vi "Type Panel Events.vi"(11 "ColumnPanel":refnum<class "ColumnPanel.lvclass">) -> (2 "Type Panel Event Reg":T1)   [LabVIEW 2020, in "Conditum-Tools.lvlib" / "ColumnPanel.lvclass"]
uses:
  ColumnPanel.lvclass
  Type Panel Event Reg.ctl
  Type Panel Events.ctl
  Conditum-Clone/Columns/Type/Type.lvclass
  ColumnPanel.lvclass/ColumnPanel.ctl
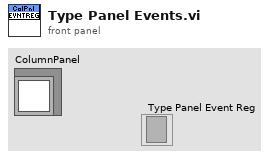
[diagram p1: front panel]
types:
  T1 = typedef "Conditum-Tools.lvlib/ColumnPanel.lvclass/Type Panel Event Reg.ctl" = refnum<event-registration>
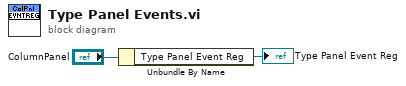
[diagram p0: block diagram]
diagram:
  n1 = Unbundle By Name("ColumnPanel") -> ("Type Panel Event Reg"=→"Type Panel Event Reg":T1)
